vi "McP Initialization.vi"(0 "VISA resource name":refnum<visa-resource-name>, 1 "error in":errorcluster) -> (2 "dup VISA Resource Name":refnum<visa-resource-name>, 3 "Initial McP Response":string, 4 "error out":errorcluster)   [LabVIEW 2019]
uses:
  Serial Instruments/Serial Support VISA.llb/Serial Actions.ctl
  Serial Instruments/Serial Support VISA.llb/Serial port parmeters.ctl
  Globals and TypeDefs/Error Categories.ctt
  <vilib>/Utility/error.llb/DialogType.ctl
panel:
  out "Final McP Response":string
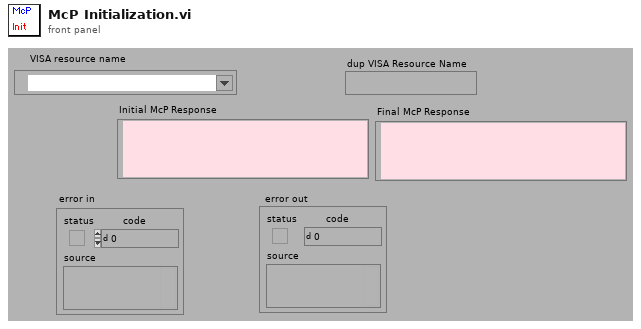
[diagram p1: front panel]
types:
  T1 = typedef "Serial Actions.ctl" = enum16{"Init", "Break", "Clear Buffer", "Write", "Read", "N Bytes", "Lock", "Unlock", "Close"}
  T2 = typedef "Serial port parmeters.ctl" = cluster{"flow control":enum16{"None", "XON/XOFF", "RTS/CTS"}, "baud rate":u32, "data bits":u16, "Stop Bits":u16, "parity (0:none)":enum16{"None", "Odd", "Even", "Mark", "Space"}, "Transmit Buffer Size":u32, "Receive Buffer Size":u32}
  T3 = enum8{"Initialization Error", "Command Error", "Parameter Error", "Overflow Error", "Time-out Error", "Misc Error", "User cancel"}
  T4 = typedef "Error Categories.ctt" = enum8{"General", "CCD-256x1024", "CCD-1340x400", "InGaAs PDA", "McPherson 2075", "Magnetic Field", "Temperature Control", "Other"}
  T5 = typedef "DialogType.ctl" = u16
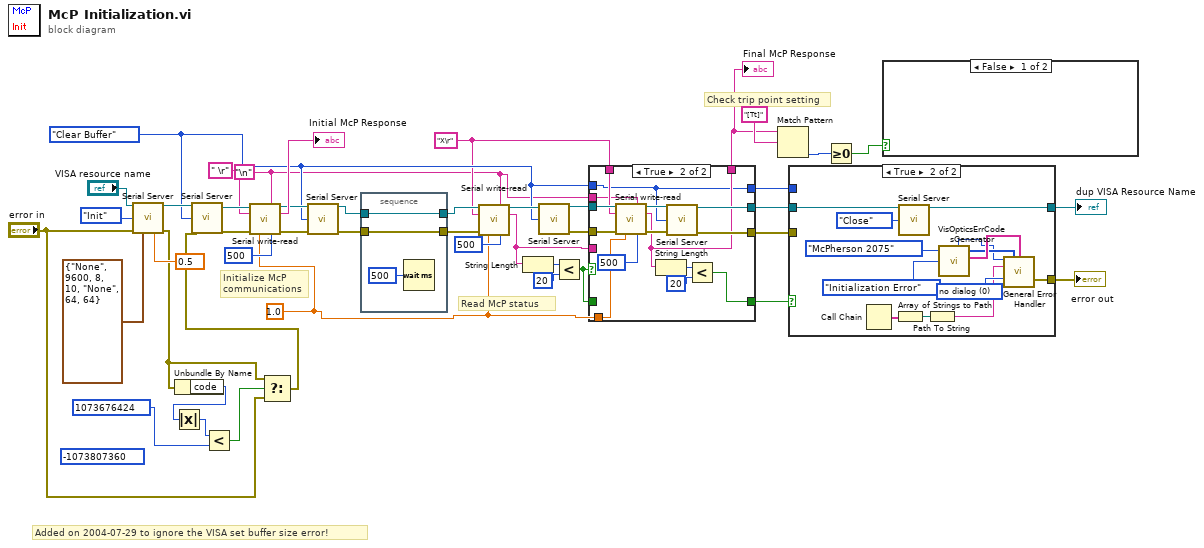
[diagram p0: block diagram]
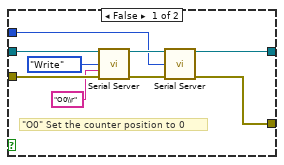
[diagram p2: hidden frame]
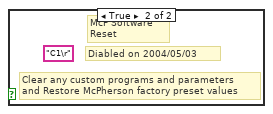
[diagram p4: hidden frame]
diagram:
  w2 = "\n"
  w3 = sgl 1.0 ("Timeout Limit(sec)")
  w6 = Serial_Actions."Clear Buffer" ("Action")
  (unwired) -1073807360 ("y")
  w5 = "X\r" ("String To Send")
  # "Added on 2004-07-29 to ignore the VISA set buffer size error!"
  # "Read McP status"
  # "Check trip point setting"
  # "Initialize McP \ncommunications"
  n1 = call "Serial Server.vi"("VISA Resource Name"="VISA resource name", "Action"=Serial_Actions."Init", "error in (no error)"="error in", "Port Parameters"=T2 {"flow control"=enum."None", "baud rate"=9600, "data bits"=8, "Stop Bits"=10, "parity (0:none)"=enum."None", "Transmit Buffer Size"=64, "Receive Buffer Size"=64}, "Timeout Limit(sec)"=0.5 ("Timeout Limit")) -> ("dup VISA Resource Name"=w36:refnum<visa-resource-name>, "error out"=w13:errorcluster)  [unwired: 6 in, 3 out]
  n2 = Unbundle By Name(w13) -> ("code"=w11:i32)
  n3 = Absolute Value(x=w11) -> (abs(x)=w10:i32)
  n4 = Less?(x=w10, y=1073676424) -> (x < y?=w9:bool)
  n5 = Select(t=w13, s=w9, f="error in") -> (s? t:f=w14:errorcluster)
  n6 = call "Serial Server.vi"("VISA Resource Name"=w36, "Action"=w6, "error in (no error)"=w14) -> ("dup VISA Resource Name"=w35:refnum<visa-resource-name>, "error out"=w38:errorcluster)  [unwired: 8 in, 3 out]
  n7 = call "Serial write-read.vi"("VISA Resource Name"=w35, "EOT Chars (cr/lf)"=w2, "String To Send"=" \r", "error in (no error)"=w38, "Timeout Limit"=w3, "milliseconds to wait"=u32 500) -> ("dup VISA Resource Name"=w31:refnum<visa-resource-name>, "Serial Read"=→"Initial McP Response":string, "error out"=w32:errorcluster)  [unwired: 4 in, 3 out]
  n8 = call "Serial Server.vi"("VISA Resource Name"=w31, "Action"=w6, "error in (no error)"=w32) -> ("dup VISA Resource Name"=w28:refnum<visa-resource-name>, "error out"=w30:errorcluster)  [unwired: 8 in, 3 out]
  n9 = stacked-sequence {
    tunnel: [w48] -> w29
    tunnel: w30 -> [w48]
    tunnel: [w46] -> w27
    tunnel: w28 -> [w46]
    frame #0 {
      n10 = Wait (ms)(milliseconds to wait=u32 500) -> ()  [unwired: 1 out]
    }
  }
  n11 = call "Serial write-read.vi"("VISA Resource Name"=w27, "EOT Chars (cr/lf)"=w2, "String To Send"=w5, "error in (no error)"=w29, "Timeout Limit"=w3, "milliseconds to wait"=u32 500) -> ("dup VISA Resource Name"=w26:refnum<visa-resource-name>, "Serial Read"=w22:string)  [unwired: 4 in, 4 out]
  n12 = String Length(string=w22) -> (length=w40:i32)
  n13 = call "Serial Server.vi"("VISA Resource Name"=w26, "Action"=w6) -> ("dup VISA Resource Name"=w25:refnum<visa-resource-name>, "error out"=w24:errorcluster)  [unwired: 9 in, 3 out]
  n14 = Less?(x=w40, y=20) -> (x < y?=w23:bool)
  n15 = case shown="True" w23 {
    tunnel: w24 -> [w52 w68]
    tunnel: w25 -> [w51 w67]
    tunnel: w6 -> [w49 w56]
    tunnel: w5 -> [_ w66]
    tunnel: [w53 w61] -> w21
    tunnel: w23 -> [w53 _]
    tunnel: [w52 w60] -> w20
    tunnel: [w51 w59] -> w19
    tunnel: w22 -> [w50 _]
    tunnel: [w50 w57] -> w16
    tunnel: [w49 w56] -> w12
    tunnel: w3 -> [_ w55]
    tunnel: w2 -> [_ w54]
    frame False {
    }
    frame True {
      n16 = call "Serial write-read.vi"("VISA Resource Name"=w67, "EOT Chars (cr/lf)"=w54, "String To Send"=w66, "error in (no error)"=w68, "Timeout Limit"=w55, "milliseconds to wait"=u32 500) -> ("dup VISA Resource Name"=w64:refnum<visa-resource-name>, "Serial Read"=w57:string, "error out"=w65:errorcluster)  [unwired: 4 in, 3 out]
      n17 = String Length(string=w57) -> (length=w63:i32)
      n18 = call "Serial Server.vi"("VISA Resource Name"=w64, "Action"=w56, "error in (no error)"=w65) -> ("dup VISA Resource Name"=w59:refnum<visa-resource-name>, "error out"=w60:errorcluster)  [unwired: 8 in, 3 out]
      n19 = Less?(x=w63, y=20) -> (x < y?=w61:bool)
    }
  }
  "Final McP Response" <- w16
  n20 = Match Pattern(string=w16, regular expression="[Tt]") -> (offset past match=w42:i32)  [unwired: 1 in, 3 out]
  n21 = case shown="True" w21 {
    tunnel: [w72 w85] -> w17
    tunnel: w20 -> [w77 _]
    tunnel: w19 -> [w76 w79]
    tunnel: [w73 w78] -> w18
    tunnel: w12 -> [w71 _]
    frame False {
      # "\"O0\" Set the counter position to 0"
      n22 = call "Serial Server.vi"("VISA Resource Name"=w76, "Action"=Serial_Actions."Write", "String To Send"="O0\\r", "error in (no error)"=w77) -> ("dup VISA Resource Name"=w74:refnum<visa-resource-name>, "error out"=w75:errorcluster)  [unwired: 7 in, 3 out]
      n23 = call "Serial Server.vi"("VISA Resource Name"=w74, "Action"=w71, "error in (no error)"=w75) -> ("dup VISA Resource Name"=w73:refnum<visa-resource-name>, "error out"=w72:errorcluster)  [unwired: 8 in, 3 out]
    }
    frame True {
      w90 = T5 0 items=["no dialog", "OK message", "continue or stop message", "OK message + warnings", "continue/stop + warnings"] ("type of dialog (OK msg:1)")
      n24 = Call Chain() -> (call chain=w83:string[])
      n25 = Array of Strings to Path(0:w83) -> (2:w82:path)  [unwired: 1 in]
      n26 = call "Serial Server.vi"("VISA Resource Name"=w79, "Action"=Serial_Actions."Close") -> ("dup VISA Resource Name"=w78:refnum<visa-resource-name>)  [unwired: 9 in, 4 out]
      n27 = Path To String(path=w82) -> (string=w81:string)
      n28 = call "VisOpticsErrCodesGenerator.vi"("NHMFL Visible Optics Error Type"=T3."Initialization Error", "NHMFL Visible Optics Error Categories"=Error_Categories.ctt."McPherson 2075") -> ("user-defined descriptions"=w89:string[], "User-defined Error Code"=w84:i32, "user-defined codes"=w88:i32[])  [unwired: 1 in, 3 out]
      n29 = call <vilib>:"General Error Handler.vi"("[error code] (0)"=w84, "[user-defined codes]"=w88, "[user-defined descriptions]"=w89, "[error source] (\" \")"=w81, "type of dialog (OK msg:1)"=w90) -> ("error out"=w85:errorcluster)  [unwired: 6 in, 4 out]
    }
  }
  "error out" <- w17
  "dup VISA Resource Name" <- w18
  n30 = Greater Or Equal To 0?(x=w42) -> (x >= 0?=w41:bool)
  n31 = case shown="False" w41 {
    frame False {
    }
    frame True {
      (unwired) "C1\r" ("String To Send")
      # "McP Software \nReset"
      # "Diabled on 2004/05/03"
      # "Clear any custom programs and parameters\nand Restore McPherson factory preset values"
    }
  }
